vi "fake THz module.vi"(10 "Main controller mailbox":T5, 11 "THz module mailbox":T5) -> ()   [LabVIEW 2021, in "THz source modeule.lvlib"]
uses:
  THz source modeule.lvlib
  Messenger service/Data types/Mailbox address.ctl
  ctl/VDI config constants.ctl
  ctl/Synth configs.ctl
  ctl/VDI status.ctl
  ctl/Synth status.ctl
  Messenger service/Data types/Module name.ctl
  ctl/THz sweep parameters.ctl
  ctl/THz Message for module.ctl
  ctl/THz commands enum.ctl
  <vilib>/ErrorRing/Error Ring.xnode
  Messenger service/MessengerLib.lvlib
panel:
  in  "Status in":T1={"Master"={"Mode"=enum."CW", "Conected"=TRUE}, "Follower"={"Mode"=enum."CW", "Conected"=TRUE}}
  out "Ended":bool
  out "?":T3={"Master"={"Lower limit [GHz]"=9.0, "Upper limit [GHz]"=15.0, "Name"="VDIS0122", "Handle"=0, "Description"="VDI Synth"}, "Follower"={"Lower limit [GHz]"=9.0, "Upper limit [GHz]"=15.0, "Name"="VDIYT7", "Handle"=0, "Description"="VDI Tracking"}}
  out "Initialized":bool
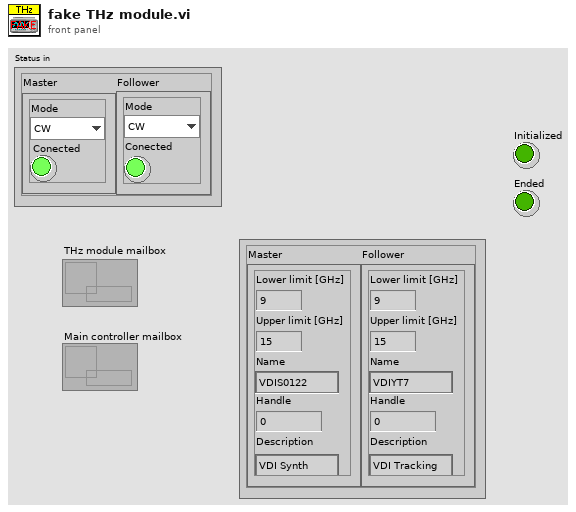
[diagram p1: front panel]
types:
  T1 = typedef "THz source modeule.lvlib/VDI status.ctl" = cluster{"Master":T2, "Follower":T2}
  T2 = typedef "THz source modeule.lvlib/Synth status.ctl" = cluster{"Mode":enum16{"CW", "Sweep"}, "Conected":bool}
  T3 = typedef "VDI config constants.ctl" = cluster{"Master":T4, "Follower":T4}
  T4 = typedef "THz source modeule.lvlib/Synth configs.ctl" = cluster{"Lower limit [GHz]":dbl, "Upper limit [GHz]":dbl, "Name":string, "Handle":u32, "Description":string}
  T5 = typedef "MessengerLib.lvlib/Mailbox address.ctl" = refnum<queue>
  T6 = typedef "Module name.ctl" = enum16{"Emty", "Magnet", "VTI", "Excitation", "Servo", "Acquisition", "Rotator", "Digitizer", "SMU2450", "Carousel", "Multimeter", "Tmp monitor", "Power monitor"}
  T7 = typedef "THz source modeule.lvlib/THz sweep parameters.ctl" = cluster{"Start [GHz]":dbl, "End [GHz] ":dbl, "Sweep up\ntime [ms]":dbl, "Sweep down\ntime [ms]":dbl, "Intermidiate [MHz]":dbl, "Reset trigger":bool}
  T8 = typedef "THz source modeule.lvlib/THz commands enum.ctl" = enum16{"Ignore", "Initialize", "Update", "Set parameters", "Disconnect", "End"}
  T9 = typedef "THz source modeule.lvlib/THz Message for module.ctl" = cluster{"Command":T8, "Data":variant}
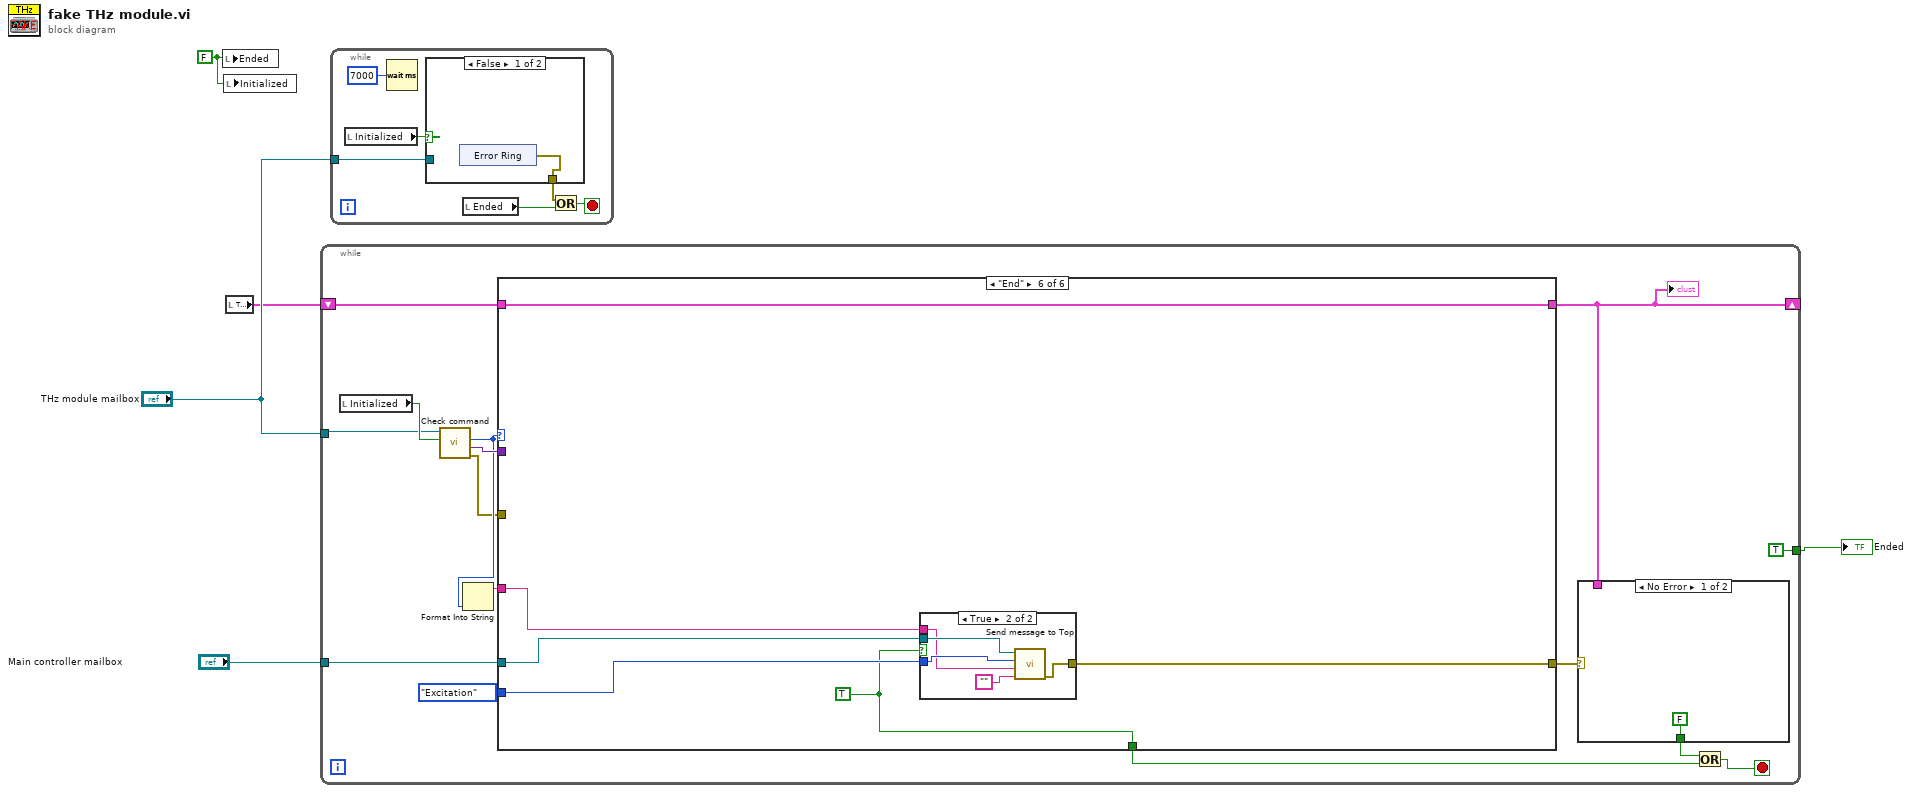
[diagram p0: block diagram]
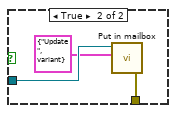
[diagram p2: hidden frame]
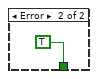
[diagram p3: hidden frame]
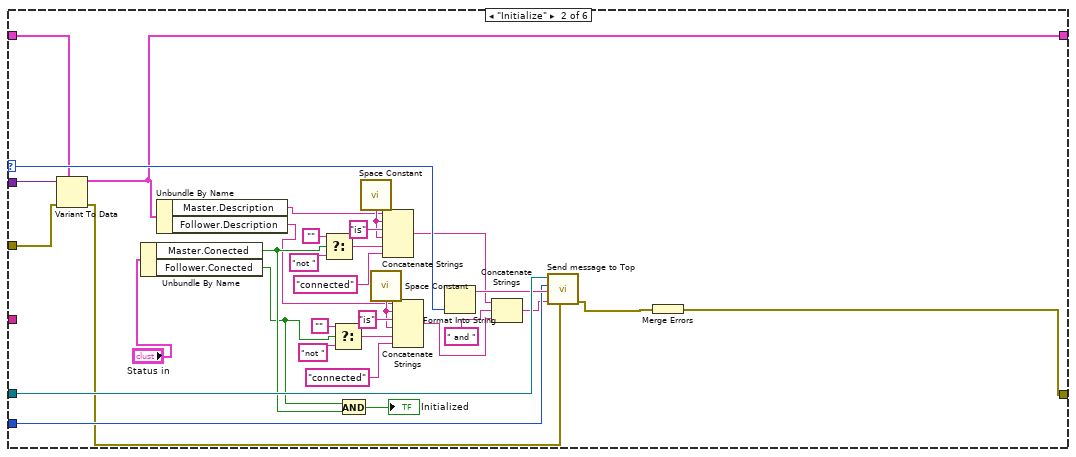
[diagram p5: hidden frame]
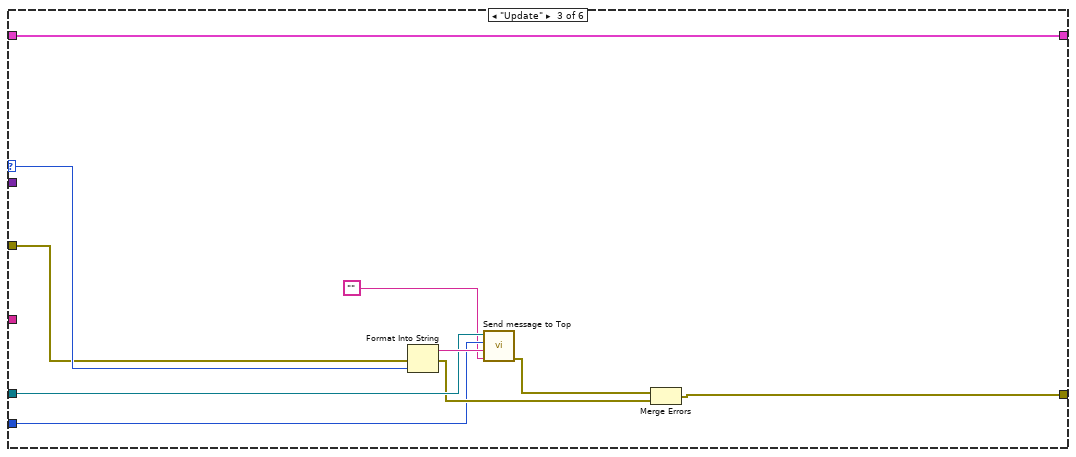
[diagram p6: hidden frame]
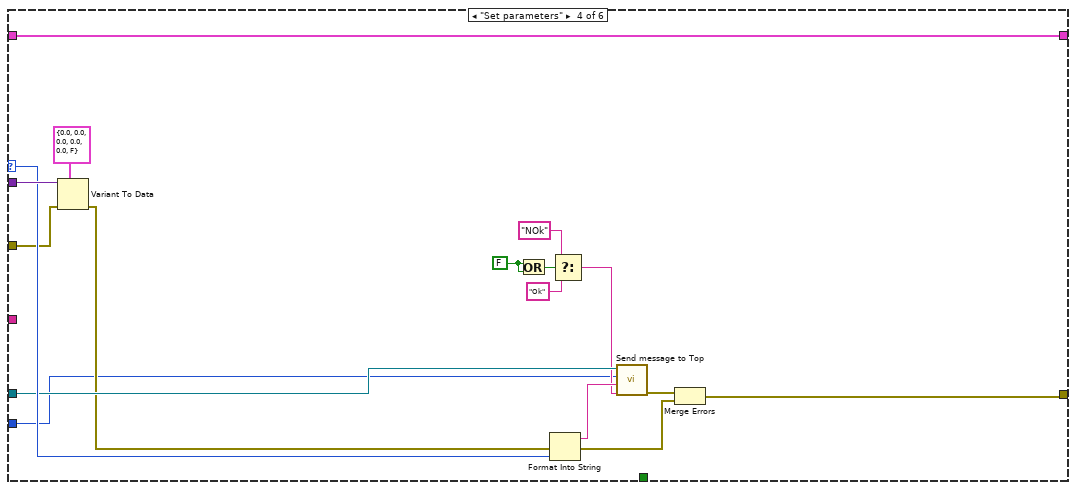
[diagram p7: hidden frame]
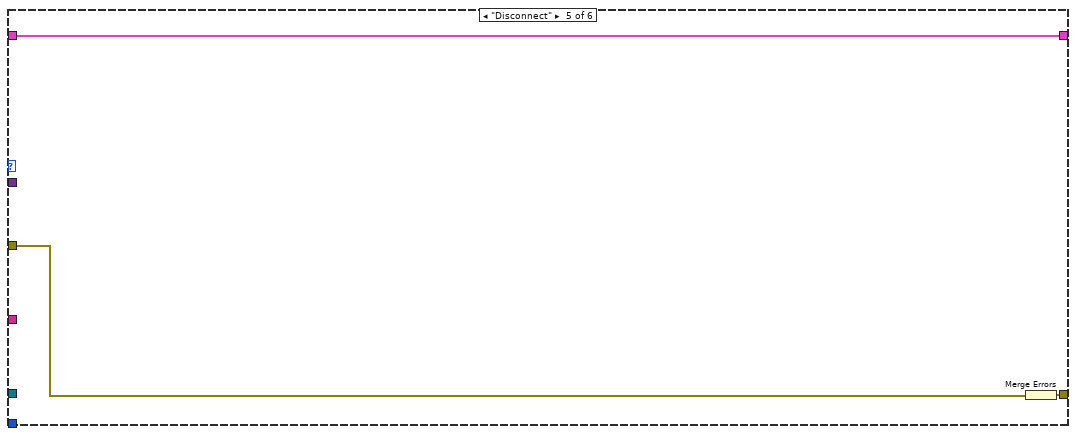
[diagram p8: hidden frame]
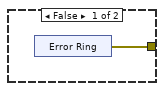
[diagram p9: hidden frame]
diagram:
  w1 = FALSE ("Initialized")
  n1 = local write "Ended"(w1) -> ()
  n2 = local write "Initialized"(w1) -> ()
  n3 = local read item#3() -> (w3:T3)
  n4 = while {
    shift-right: [w16] -> _
    shift-left: w3 -> [w20]
    tunnel: "THz module mailbox" -> [w7]
    tunnel: "Main controller mailbox" -> [w19]
    tunnel: [TRUE ("Initialized")] -> w2
    stop <- w14 stop-if-true
    n5 = local read "Initialized"() -> (w17:bool)
    n6 = call "Check command.vi"("Is initialized"=w17, "Module mailbox"=w7) -> ("error out"=w6:errorcluster, "Command Data"=w18:variant, "Command"=w9:T8)  [unwired: 3 in]
    n7 = Format Into String(w9) -> (resulting string=w8:string)  [unwired: 3 in, 1 out]
    n8 = case shown="\"End\"" w9 {
      selector: w9 -> [_ w45 w66 w80 _ _]
      tunnel: [w24 w29 w60 w83 w87 w89] -> w16
      tunnel: w20 -> [w24 w36 w60 w83 w87 w89]
      tunnel: w18 -> [_ w57 _ w84 _ _]
      tunnel: [_ _ _ _ _ w88] -> w15
      tunnel: w19 -> [_ w44 w65 w79 _ w93]
      tunnel: [w23 w40 w63 w72 w85 w92] -> w11
      tunnel: w6 -> [w23 w38 w62 w74 w86 _]
      tunnel: Module_name."Excitation" ("Module") -> [_ w31 w59 w69 _ w91]
      tunnel: w8 -> [_ _ _ _ _ w90]
      frame "Ignore", Default {
      }
      frame "Initialize" {
        n9 = Variant To Data(error in=w38, type=w36, Variant=w57) -> (data=w29:T3, error out=w25:errorcluster)
        n10 = Unbundle By Name("Status in") -> ("Master.Conected"=w41:bool, "Follower.Conected"=w32:bool)
        n11 = Unbundle By Name(w29) -> ("Master.Description"=w34:string, "Follower.Description"=w33:string)
        n12 = Select(t="", s=w41, f="not ") -> (s? t:f=w53:string)
        n13 = Select(t="", s=w32, f="not ") -> (s? t:f=w49:string)
        n14 = And(x=w32, y=w41) -> (x .and. y?=→"Initialized":bool)
        n15 = call <vilib>:"Space Constant.vi"() -> ("String"=w52:string)
        n16 = call <vilib>:"Space Constant.vi"() -> ("String"=w37:string)
        n17 = Concatenate Strings(w34, w52, "is", w52, w53, "connected") -> (w35:string)
        n18 = Concatenate Strings(w33, w37, "is", w37, w49, "connected") -> (w27:string)
        n19 = Format Into String(w45) -> (resulting string=w43:string)  [unwired: 3 in, 1 out]
        n20 = Concatenate Strings(w35, " and ", w27) -> (w28:string)
        n21 = call "Send message to Top.vi"("Error in (no error)"=w25, "Data"=w28, "Response"=w43, "Module"=w31, "Mailbox address in"=w44) -> ("Error out"=w39:errorcluster)  [unwired: 5 in, 1 out]
        n22 = Merge Errors(w39) -> (w40:errorcluster)
      }
      frame "Update" {
        n23 = Format Into String(error in=w62, w66) -> (resulting string=w67:string, error out=w61:errorcluster)  [unwired: 2 in]
        n24 = call "Send message to Top.vi"("Data"="", "Response"=w67, "Module"=w59, "Mailbox address in"=w65) -> ("Error out"=w64:errorcluster)  [unwired: 6 in, 1 out]
        n25 = Merge Errors(w64, w61) -> (w63:errorcluster)
      }
      frame "Set parameters" {
        w68 = FALSE ("x")
        n26 = Variant To Data(error in=w74, type=T7 {"Start [GHz]"=0.0, "End [GHz] "=0.0, "Sweep up\ntime [ms]"=0.0, "Sweep down\ntime [ms]"=0.0, "Intermidiate [MHz]"=0.0, "Reset trigger"=FALSE} ("Sweep parameters"), Variant=w84) -> (error out=w73:errorcluster)  [unwired: 1 out]
        n27 = Or(x=w68, y=w68) -> (x .or. y?=w78:bool)
        n28 = Format Into String(error in=w73, w80) -> (resulting string=w81:string, error out=w71:errorcluster)  [unwired: 2 in]
        n29 = Select(t="NOk", s=w78, f="Ok") -> (s? t:f=w76:string)
        n30 = call "Send message to Top.vi"("Data"=w76, "Response"=w81, "Module"=w69, "Mailbox address in"=w79) -> ("Error out"=w70:errorcluster)  [unwired: 6 in, 1 out]
        n31 = Merge Errors(w70, w71) -> (w72:errorcluster)
      }
      frame "Disconnect" {
        n32 = Merge Errors(w86) -> (w85:errorcluster)
      }
      frame "End" {
        w88 = TRUE
        n33 = case shown="True" w88 {
          tunnel: w93 -> [_ w100]
          tunnel: [w94 w99] -> w92
          tunnel: w91 -> [_ w97]
          tunnel: w90 -> [_ w96]
          frame False {
            n34 = xnode "Error Ring"() -> ("error out"=w94:errorcluster)
          }
          frame True {
            n35 = call "Send message to Top.vi"("Data"="", "Response"=w96, "Module"=w97, "Mailbox address in"=w100) -> ("Error out"=w99:errorcluster)  [unwired: 6 in, 1 out]
          }
        }
      }
    }
    "?" <- w16
    n36 = case shown="No Error" w11 {
      tunnel: w16 -> [_ _]
      tunnel: [FALSE TRUE] -> w13
      frame No Error {
      }
      frame Error {
      }
    }
    n37 = Or(x=w13, y=w15) -> (x .or. y?=w14:bool)
  }
  "Ended" <- w2
  n38 = while {
    tunnel: "THz module mailbox" -> [w104]
    stop <- w103 stop-if-true
    n39 = local read "Initialized"() -> (w105:bool)
    n40 = Wait (ms)(milliseconds to wait=u32 7000) -> ()  [unwired: 1 out]
    n41 = case shown="False" w105 {
      tunnel: w104 -> [_ w111]
      tunnel: [w107 w109] -> w102
      frame False {
        n42 = xnode "Error Ring"() -> ("error out"=w107:errorcluster)
      }
      frame True {
        n43 = call "Put in mailbox.vi"("Message"=T9 {"Command"=enum."Update", "Data"=variant} ("Incoming msg"), "Queue in"=w111) -> ("error out"=w109:errorcluster)  [unwired: 7 in, 2 out]
      }
    }
    n44 = local read "Ended"() -> (w101:bool)
    n45 = Or(x=w102, y=w101) -> (x .or. y?=w103:bool)
  }
